vi "Get ADC.vi"(5 "Gain":u16(ring) items=["High", "Med", "Low"], 7 "Detector":u16(ring) items=["SWIR", "MWIR"], 8 "error in (no error)":errorcluster, 11 "VISA resource name":refnum<visa-resource-name>) -> (0 "error out":errorcluster, 2 "output":i32, 3 "VISA resource name out":refnum<visa-resource-name>)   [LabVIEW 2025, in "Detector SCPI.lvlib"]
doc: "Read ADC channel from detector board\n\nChannel is 0..7\nReturns integer value after oversampling, if any"
uses:
  Detector SCPI.lvlib
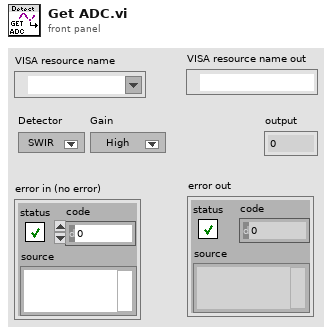
[diagram p1: front panel]
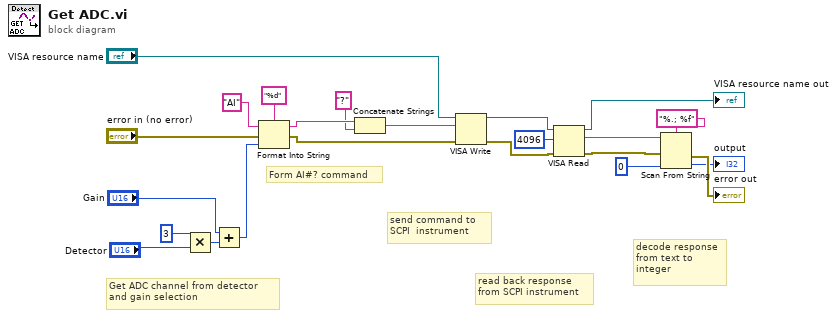
[diagram p0: block diagram]
diagram:
  # "decode response\nfrom text to\ninteger"
  # "read back response\nfrom SCPI instrument"
  # "send command to \nSCPI  instrument"
  # "Form AI#? command"
  # "Get ADC channel from detector \nand gain selection"
  n1 = Multiply(x=u16 3, y="Detector") -> (x*y=w4:u16)
  n2 = Add(x="Gain", y=w4) -> (x+y=w1:u16)
  n3 = Format Into String(format string="%d", initial string="AI" ("command"), error in="error in (no error)", w1) -> (resulting string=w16:string, error out=w22:errorcluster)
  n4 = Concatenate Strings(w16, "?" ("command")) -> (w17:string)
  n5 = VISA Write(VISA resource name="VISA resource name", write buffer=w17, error in (no error)=w22) -> (VISA resource name out=w6:refnum<visa-resource-name>, error out=w18:errorcluster)  [unwired: 1 out]
  n6 = VISA Read(VISA resource name=w6, byte count=u32 4096, error in (no error)=w18) -> (VISA resource name out=→"VISA resource name out":refnum<visa-resource-name>, read buffer=w12:string, error out=w10:errorcluster)  [unwired: 1 out]
  n7 = Scan From String(format string="%.; %f", input string=w12, error in=w10, default 1=0 ("default value 1")) -> (error out=→"error out":errorcluster, output 1=→"output":i32)  [unwired: 1 in, 2 out]
